vi "Write Input Registers.vi"(8 "error in (no error)":errorcluster, 9 "register values":u16[](array[numeric]), 10 "starting address":u16, 11 "standard data model in":refnum<class "ICPCON ET Data Model.lvclass">) -> (0 "error out":errorcluster, 3 "standard data model out":refnum<class "ICPCON ET Data Model.lvclass">)   [LabVIEW 2021, in "ICPCON ET Data Model.lvclass"]
doc: "Writes the values of multiple input register values in series, starting at address M."
uses:
  ICPCON ET Data Model.lvclass
  ICPCON ET Data Model.lvclass/ICPCON ET Data Model.ctl
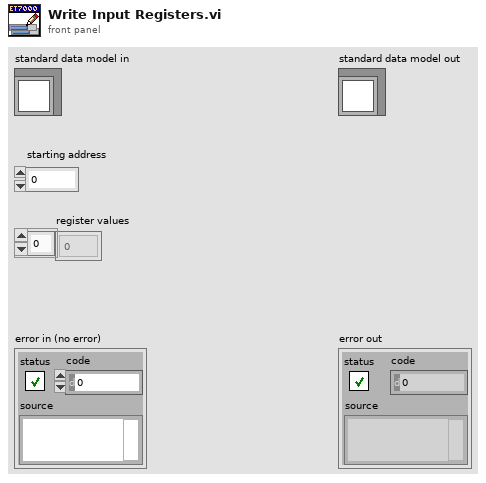
[diagram p1: front panel]
types:
  T1 = typedef "ICPCON ET Data Model.lvclass/Data Model.ctl" = cluster{"UTC":u64, "DI":bool[], "DO":bool[], "IR":u16[], "HR":u16[], "ES":u8}
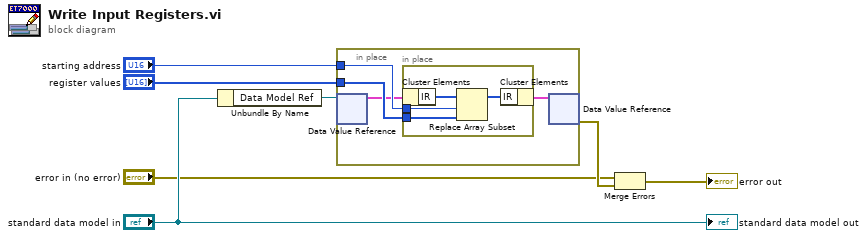
[diagram p0: block diagram]
diagram:
  n1 = Unbundle By Name("standard data model in") -> ("Data Model Ref"=w3:refnum<data-value>)
  n2 = in-place {
    in-place-border: "starting address" -> [w11]
    in-place-border: "register values" -> [w10]
    n3 = in-place-dvr #1(w3) -> (w9:T1)  [unwired: 1 out]
    n4 = in-place {
      in-place-border: w11 -> [w15]
      in-place-border: w10 -> [w14]
      n5 = in-place-cluster #2(w9) -> ("IR"=w13:u16[])
      n6 = Replace Array Subset(array=w13, new element=w14, index=w15) -> (w12:u16[])
      n7 = in-place-cluster #2("IR"=w12) -> (w8:T1)
    }
    n8 = in-place-dvr #1(w8) -> (w2:errorcluster)  [unwired: 1 out]
  }
  n9 = Merge Errors("error in (no error)", w2) -> (→"error out":errorcluster)
  "standard data model out" <- "standard data model in"
